vi "HTVacuumGUI.panel.vi"(0 "object ref":refnum<vi>, 5 "error in (no error)":errorcluster) -> (19 "error out":errorcluster)   [LabVIEW 2014, in "HTVacuumGUI.lvlib"]
doc: "This is just an example for a GUI thread.\n\nLicense Agreement for this software:\n\nCopyright (C)\nGesellschaft für Schwerionenforschung, GSI\nPlanckstr. 1\n64291 Darmstadt\nGermany\n\nContact: D.Beck@gsi.de \n\nThis program is free software; you can redistribute it and/or modify it under the terms of the GNU General Public License as published by the Free Software Foundation; either version 2 of the license, or (at your option) any later version.\n\nThis program is distributed in the hope that it will be useful, but WITHOUT ANYW ARRANTY; without even the implied warranty of MERCHANTABILITY or FITNESS FOR A PARTICULAR PURPOSE. See the GNU General License for more details (http://www.gnu.org).\n\nGesellschaft für Schwerionenforschung, GSI\nPlanckstr. 1, 64291 Darmstadt, Germany\nFor all questions and ideas contact: M.Richter@gsi.de, H.Brand@gsi.de or D.Beck@gsi.de.\nLast update: 18-DEC-2002"
uses:
  HTVacuumGUI.lvlib
  CS_Core/CSSystem/CoreLib/CoreLib.int 2 byte array.vi
  CS_Core/CSSystem/CoreLib/CoreLib.byte array 2 int.vi
  CS_Core/CSSystem/CoreLib/CoreLib.byte array 2 short.vi
  CS_Core/BaseProcess/BaseProcess.lvlib
  CS_Core/GUIs/GOGUserGUIs/DeviceBaseGUI/DeviceBaseGUI.lvlib
  CS_Core/CSSystem/CoreLib/CoreLib.lvlib
  CS_Core/CSSystem/CSSystemLib/CSSystemLib.lvlib
  CS_Core/CSObj/CSObj.lvlib
panel:
  in  "V62":bool
  out "V62":u32(colorbox)
  in  "V61":bool
  out "V61":u32(colorbox)
  in  "V52":bool
  out "V52":u32(colorbox)
  in  "V71":bool
  out "V71":u32(colorbox)
  in  "V1":bool
  out "V1":u32(colorbox)
  in  "VP3":bool
  out "VP3":u32(colorbox)
  in  "VP2":bool
  out "VP2":u32(colorbox)
  in  "VP1":bool
  out "VP1":u32(colorbox)
  in  "P3":bool
  out "P3":u32(colorbox)
  in  "P2":bool
  out "P2":u32(colorbox)
  in  "P1":bool
  out "P1":u32(colorbox)
  in  "SG 3VL":bool caption="Blank Button"
  in  "SG 2VL":bool caption="Blank Button"
  in  "SG 1VL":bool caption="Blank Button"
  in  "SG 3L":bool caption="Blank Button"
  in  "SG 2L":bool caption="Blank Button"
  in  "SG 1L":bool caption="Blank Button"
  in  "SP 3":bool caption="Blank Button"
  in  "SP 2":bool caption="Blank Button"
  out "G3":dbl(slide) scale=0.0..2.0
  out "G2":dbl(slide) scale=0.0..2.0
  out "G1":dbl(slide) scale=0.0..2.0
  in  "SP 1":bool caption="Blank Button"
  in  "stop":bool
  out "loop counter":i32
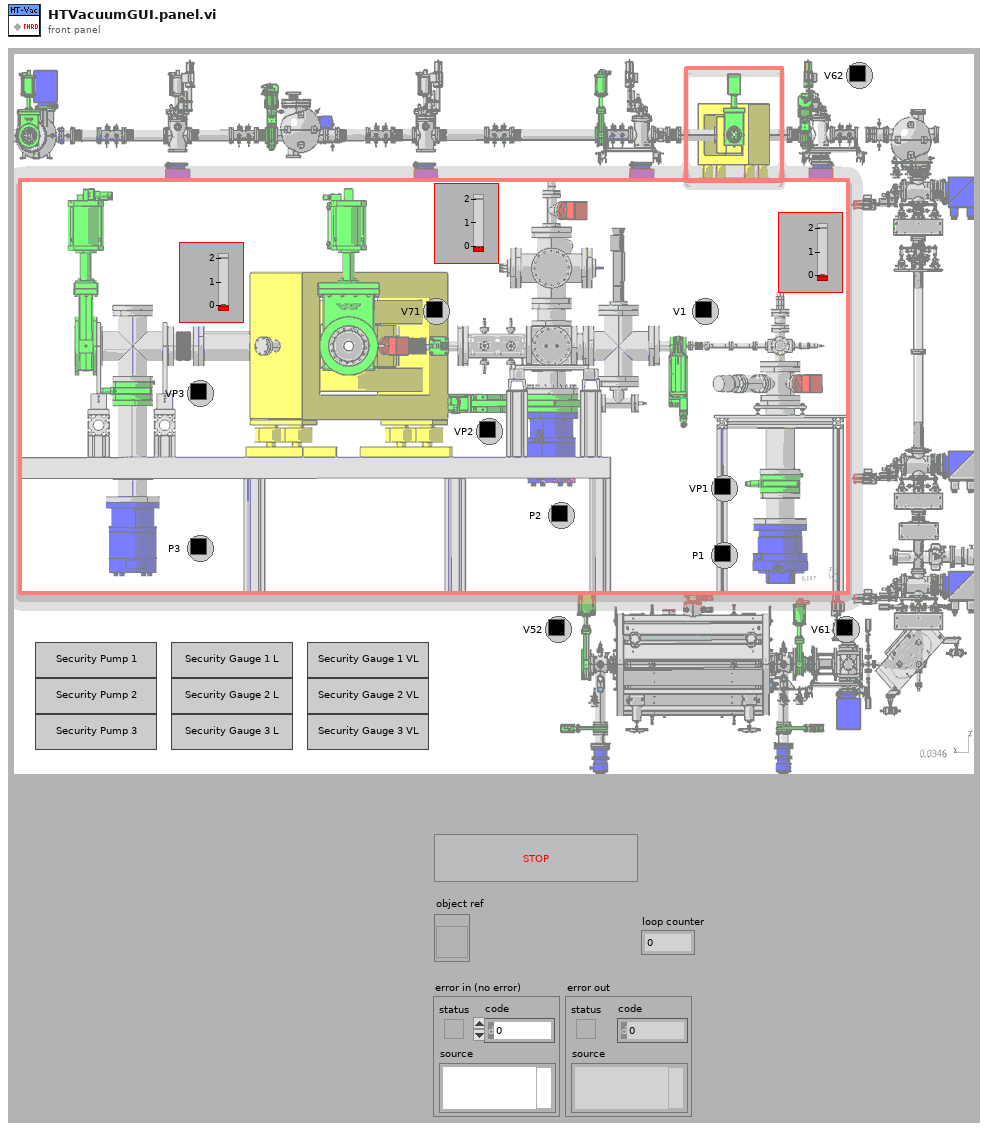
[diagram p1: front panel]
types:
  T1 = typedef "Semaphore RefNum" = refnum<k1>
  T2 = typedef "CoreDefs.rawDataType.ctl" = i8[]
  T3 = typedef "CoreDefs.call_type.ctl" = cluster{"Object":string, "Selector":string, "CallType":enum16{"simple", "synchronous", "asynchronous"}, "Async Object":string, "Async Selector":string, "Data Descriptor":T4, "Data":T2, "Error #":i32, "Expire":u32}
  T4 = typedef "BaseProcess.lvlib/BaseProcess.descriptor string definition.ctl" = string
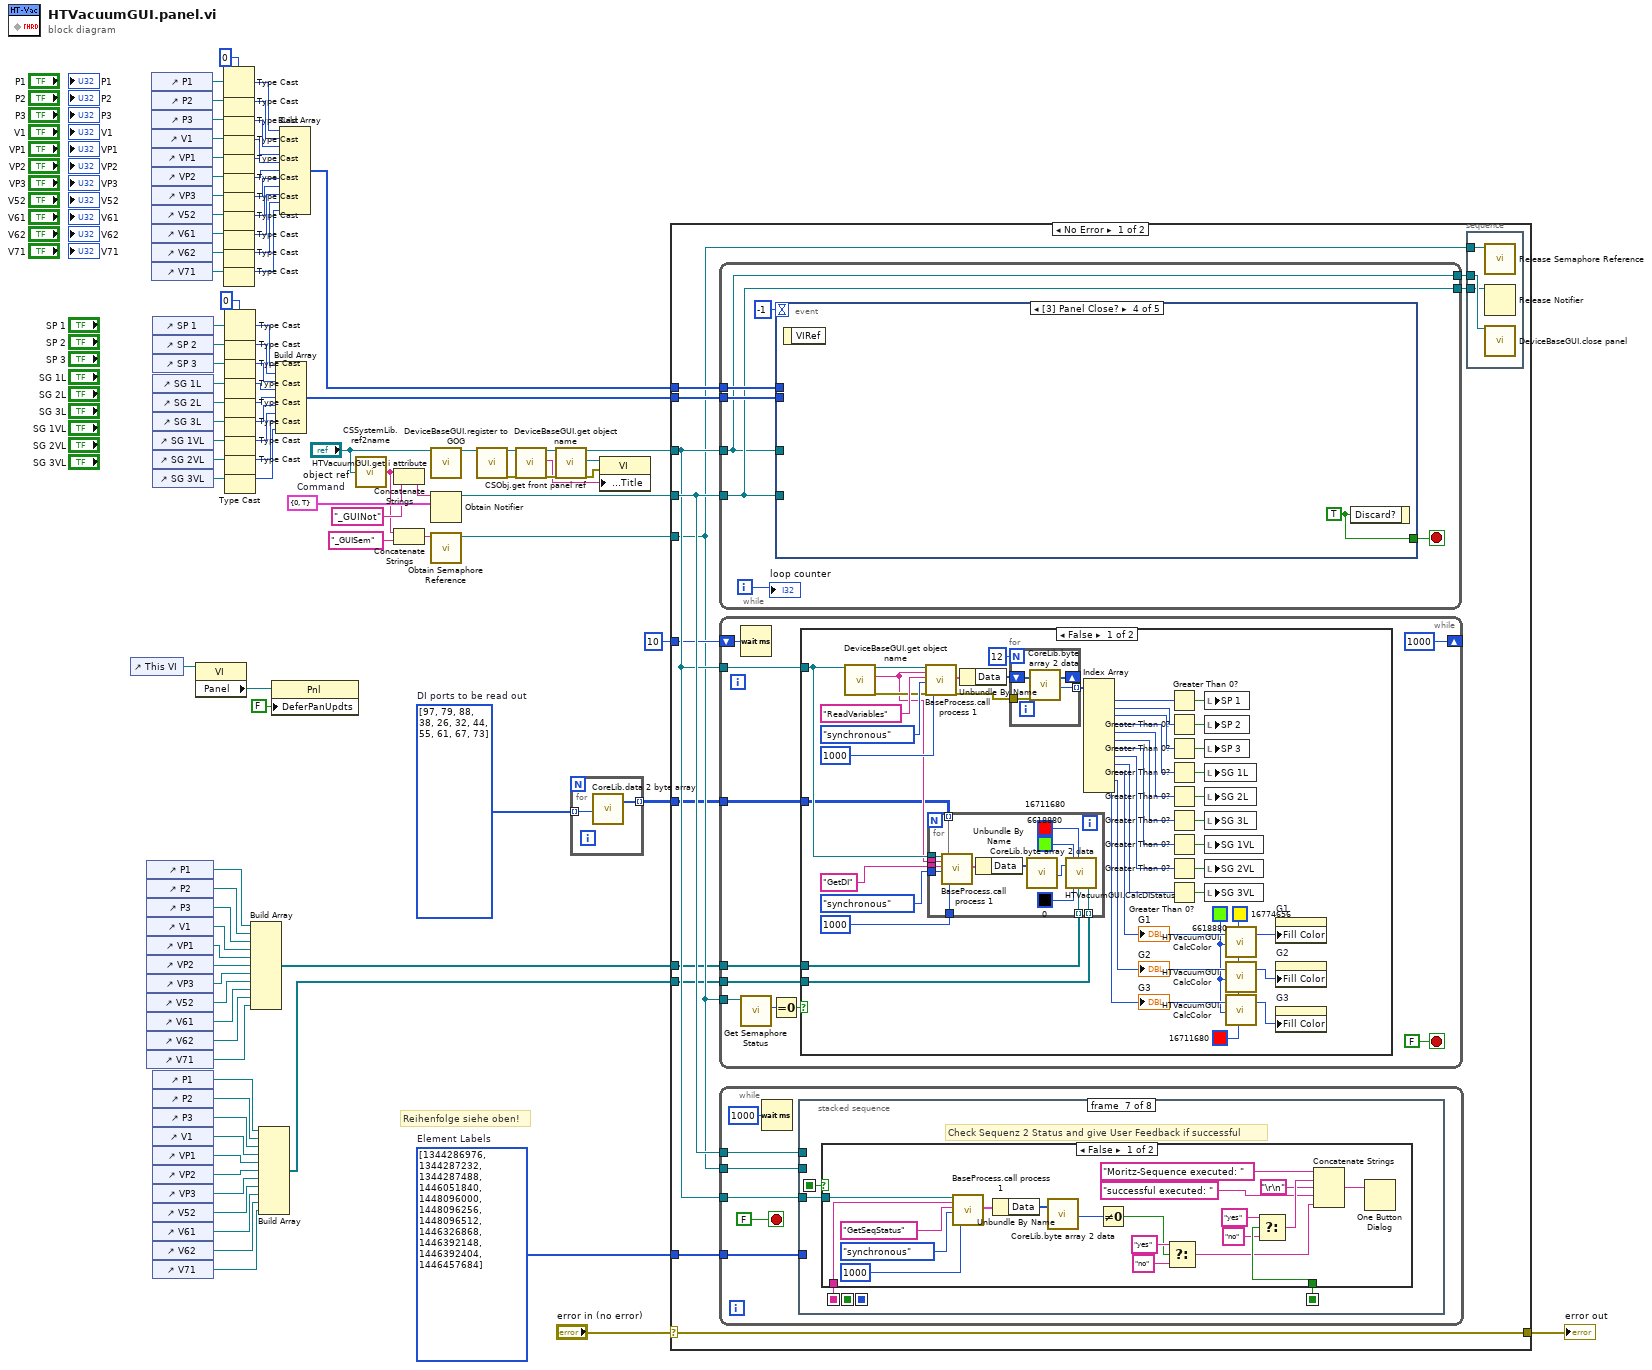
[diagram p0: block diagram]
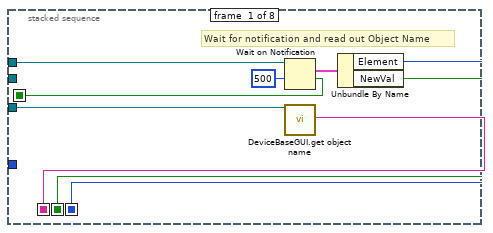
[diagram p2: hidden frame]
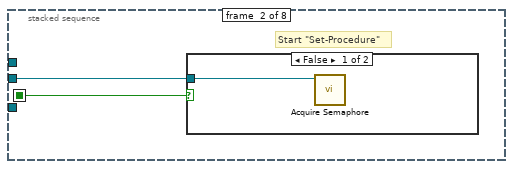
[diagram p3: hidden frame]
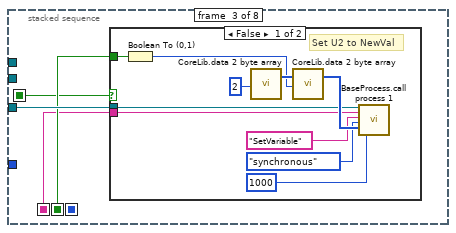
[diagram p5: hidden frame]
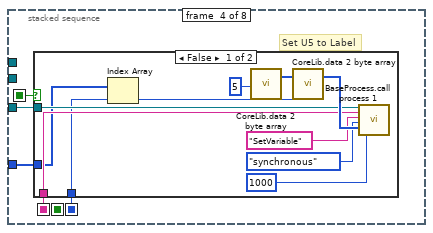
[diagram p7: hidden frame]
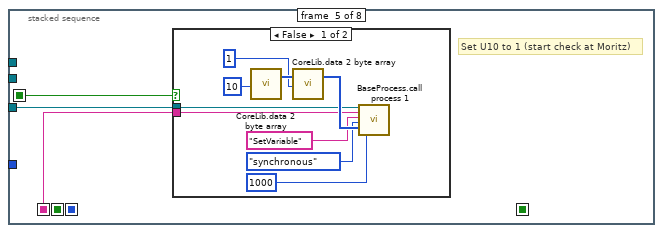
[diagram p9: hidden frame]
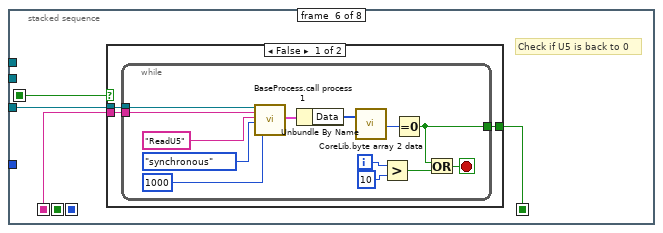
[diagram p11: hidden frame]
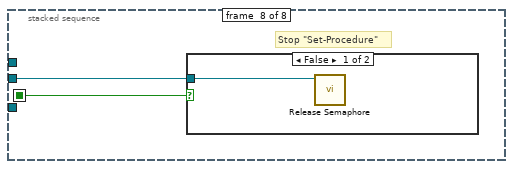
[diagram p14: hidden frame]
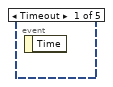
[diagram p17: hidden frame]
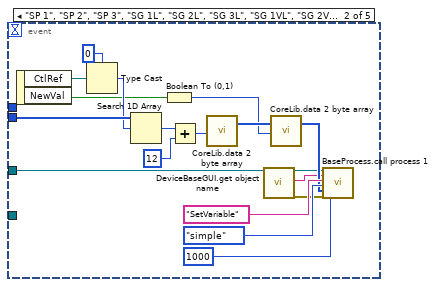
[diagram p18: hidden frame]
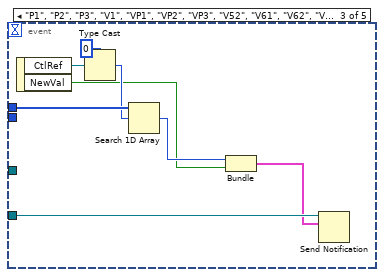
[diagram p19: hidden frame]
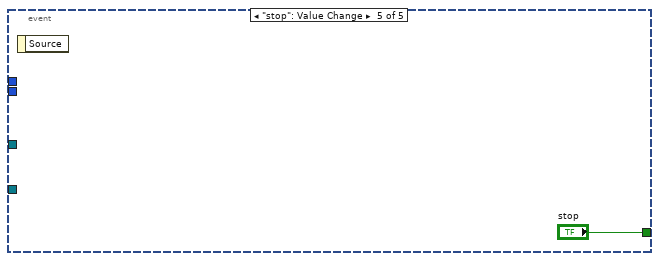
[diagram p20: hidden frame]
diagram:
  w29 = i32[] [97, 79, 88, 38, 26, 32, 44, 55, 61, 67, 73]  # DI ports to be read out
  w44 = i32[] [1344286976, 1344287232, 1344287488, 1446051840, 1448096000, 1448096256, 1448096512, 1446326868, 1446392148, 1446392404, 1446457684]  # Element Labels
  w49 = cluster{"Element":i32, "NewVal":bool} {"Element"=0, "NewVal"=TRUE}  # Command
  w51 = 0
  w84 = 0
  # "Reihenfolge siehe oben!"
  n1 = control-ref of="This VI"() -> (w3:refnum<vi>)
  n2 = control-ref of="P1"() -> (w27:refnum<vi>)
  n3 = control-ref of="P2"() -> (w26:refnum<vi>)
  n4 = control-ref of="P3"() -> (w25:refnum<vi>)
  n5 = control-ref of="V1"() -> (w24:refnum<vi>)
  n6 = control-ref of="VP1"() -> (w23:refnum<vi>)
  n7 = control-ref of="VP2"() -> (w22:refnum<vi>)
  n8 = control-ref of="VP3"() -> (w21:refnum<vi>)
  n9 = control-ref of="V52"() -> (w20:refnum<vi>)
  n10 = control-ref of="V61"() -> (w19:refnum<vi>)
  n11 = control-ref of="V62"() -> (w18:refnum<vi>)
  n12 = control-ref of="V71"() -> (w17:refnum<vi>)
  n13 = control-ref of="P1"() -> (w64:refnum<vi>)
  n14 = control-ref of="P2"() -> (w63:refnum<vi>)
  n15 = control-ref of="P3"() -> (w62:refnum<vi>)
  n16 = control-ref of="V1"() -> (w61:refnum<vi>)
  n17 = control-ref of="VP1"() -> (w60:refnum<vi>)
  n18 = control-ref of="VP2"() -> (w59:refnum<vi>)
  n19 = control-ref of="VP3"() -> (w58:refnum<vi>)
  n20 = control-ref of="V52"() -> (w57:refnum<vi>)
  n21 = control-ref of="V61"() -> (w56:refnum<vi>)
  n22 = control-ref of="V62"() -> (w55:refnum<vi>)
  n23 = control-ref of="V71"() -> (w54:refnum<vi>)
  n24 = control-ref of="SP 1"() -> (w93:refnum<vi>)
  n25 = control-ref of="SP 2"() -> (w92:refnum<vi>)
  n26 = control-ref of="SP 3"() -> (w91:refnum<vi>)
  n27 = control-ref of="SG 1L"() -> (w90:refnum<vi>)
  n28 = control-ref of="SG 2L"() -> (w89:refnum<vi>)
  n29 = control-ref of="SG 3L"() -> (w88:refnum<vi>)
  n30 = control-ref of="SG 1VL"() -> (w87:refnum<vi>)
  n31 = control-ref of="SG 2VL"() -> (w86:refnum<vi>)
  n32 = control-ref of="SG 3VL"() -> (w85:refnum<vi>)
  n33 = control-ref of="P1"() -> (w15:refnum<vi>)
  n34 = control-ref of="P2"() -> (w14:refnum<vi>)
  n35 = control-ref of="P3"() -> (w13:refnum<vi>)
  n36 = control-ref of="V1"() -> (w12:refnum<vi>)
  n37 = control-ref of="VP1"() -> (w11:refnum<vi>)
  n38 = control-ref of="VP2"() -> (w10:refnum<vi>)
  n39 = control-ref of="VP3"() -> (w9:refnum<vi>)
  n40 = control-ref of="V52"() -> (w8:refnum<vi>)
  n41 = control-ref of="V61"() -> (w7:refnum<vi>)
  n42 = control-ref of="V62"() -> (w6:refnum<vi>)
  n43 = control-ref of="V71"() -> (w5:refnum<vi>)
  n44 = property class="VI"(reference=w3) -> ("Panel"=w2:refnum<vi>)  [unwired: 1 in, 2 out]
  n45 = Type Cast(type=w51, x=w64) -> (*(type *) &x=w73:i32)
  n46 = Type Cast(type=w51, x=w63) -> (*(type *) &x=w72:i32)
  n47 = Type Cast(type=w51, x=w62) -> (*(type *) &x=w71:i32)
  n48 = Type Cast(type=w51, x=w61) -> (*(type *) &x=w70:i32)
  n49 = Type Cast(type=w51, x=w60) -> (*(type *) &x=w69:i32)
  n50 = Type Cast(type=w51, x=w59) -> (*(type *) &x=w68:i32)
  n51 = Type Cast(type=w51, x=w58) -> (*(type *) &x=w67:i32)
  n52 = Type Cast(type=w51, x=w57) -> (*(type *) &x=w66:i32)
  n53 = Type Cast(type=w51, x=w56) -> (*(type *) &x=w65:i32)
  n54 = Type Cast(type=w51, x=w55) -> (*(type *) &x=w53:i32)
  n55 = Type Cast(type=w51, x=w54) -> (*(type *) &x=w52:i32)
  n56 = Type Cast(type=w84, x=w93) -> (*(type *) &x=w83:i32)
  n57 = Type Cast(type=w84, x=w92) -> (*(type *) &x=w82:i32)
  n58 = Type Cast(type=w84, x=w91) -> (*(type *) &x=w81:i32)
  n59 = Type Cast(type=w84, x=w90) -> (*(type *) &x=w80:i32)
  n60 = Type Cast(type=w84, x=w89) -> (*(type *) &x=w79:i32)
  n61 = Type Cast(type=w84, x=w88) -> (*(type *) &x=w78:i32)
  n62 = Type Cast(type=w84, x=w87) -> (*(type *) &x=w77:i32)
  n63 = Type Cast(type=w84, x=w86) -> (*(type *) &x=w76:i32)
  n64 = Type Cast(type=w84, x=w85) -> (*(type *) &x=w75:i32)
  n65 = Build Array(w27, w26, w25, w24, w23, w22, w21, w20, w19, w18, w17) -> (w16:refnum<vi>[])
  n66 = Build Array(w15, w14, w13, w12, w11, w10, w9, w8, w7, w6, w5) -> (w4:refnum<vi>[])
  n67 = property class="Pnl"(reference=w2, "DeferPanUpdts"=FALSE ("Defer Panel Updates")) -> ()  [unwired: 1 in, 2 out]
  n68 = Build Array(w83, w82, w81, w80, w79, w78, w77, w76, w75) -> (w74:i32[])
  n69 = Build Array(w73, w72, w71, w70, w69, w68, w67, w66, w65, w53, w52) -> (w50:i32[])
  n70 = call "CSSystemLib.ref2name.vi"("obj refnum"="object ref") -> ("name"=w42:string)
  n71 = Concatenate Strings(w42, "_GUINot" ("string")) -> (w47:string)
  n72 = Concatenate Strings(w42, "_GUISem" ("string")) -> (w43:string)
  n73 = call "HTVacuumGUI.get i attribute.vi"("i ref in"="object ref") -> ("i ref out"=w32:refnum<vi>)  [unwired: 16 in, 2 out]
  n74 = Obtain Notifier(name (unnamed)=w47, notification data type=w49) -> (notifier out=w45:refnum<notifier>)  [unwired: 2 in, 2 out]
  n75 = call <vilib>:"Obtain Semaphore Reference.vi"("name (unnamed)"=w43) -> ("semaphore"=w40:T1)  [unwired: 4 in, 2 out]
  n76 = call "DeviceBaseGUI.register to GOG.vi"("i ref in"=w32) -> ("i ref out"=w37:refnum<vi>, "error out"=w38:errorcluster)  [unwired: 16 in, 1 out]
  n77 = call "DeviceBaseGUI.get object name.vi"("i ref in"=w37, "error in (no error)"=w38) -> ("i ref out"=w36:refnum<vi>, "objectName"=w33:string, "error out"=w35:errorcluster)  [unwired: 15 in]
  n78 = call "CSObj.get front panel ref.vi"("i ref in"=w36, "error in (no error)"=w35) -> ("i ref out"=w31:refnum<vi>, "frontPanelRef"=w39:refnum<vi>, "error out"=w34:errorcluster)  [unwired: 15 in]
  n79 = for {
    tunnel: w29 -> [w97] mode=indexing
    tunnel: [w96] -> w28 mode=indexing
    n80 = call-poly "CoreLib.data 2 byte array.vi"("i32"=w97) -> ("byteArray out"=w96:T2)  [unwired: 18 in]
  }
  n81 = property class="VI"(reference=w39, error in=w34, "Front Panel Window:Title"=w33) -> ()  [unwired: 2 out]
  n82 = case shown="No Error" "error in (no error)" {
    selector: "error in (no error)" -> [w110 w331]
    tunnel: [w110 w331] -> w94
    tunnel: w31 -> [w106 w330]
    tunnel: w74 -> [w109 _]
    tunnel: w50 -> [w108 _]
    tunnel: w45 -> [w107 w328]
    tunnel: w44 -> [w105 _]
    tunnel: w40 -> [w101 w329]
    tunnel: 10 -> [w104 _]
    tunnel: w28 -> [w100 _]
    tunnel: w16 -> [w99 _]
    tunnel: w4 -> [w98 _]
    frame No Error {
      n83 = while {
        tunnel: w106 -> [w293]
        tunnel: w109 -> [w296]
        tunnel: w108 -> [w295]
        tunnel: w107 -> [w294]
        tunnel: [w294] -> w102
        tunnel: [w293] -> w103
        i -> [w298]
        stop <- w299 stop-if-true
        n84 = event shown="[3] Panel Close?" {
          selector: _ -> [_ _ _ _ _]
          dyn-events: _ -> [_ _ _ _ _]
          timeout: -1 -> [_ _ _ _ _]
          tunnel: [_ _ _ w326 "stop"] -> w299
          tunnel: w293 -> [_ w301 _ _ _]
          tunnel: w296 -> [_ w315 _ _ _]
          tunnel: w295 -> [_ _ w323 _ _]
          tunnel: w294 -> [_ _ w321 _ _]
          event Timeout {
            n85 = event-data() -> ()  [unwired: 1 in, 1 out]
          }
          event "SP 1", "SP 2", "SP 3", "SG 1L", "SG 2L", "SG 3L", "SG 1VL", "SG 2VL", "SG 3VL": Value Change {
            n86 = event-data() -> ("CtlRef"=w316:refnum<vi>, "NewVal"=w308:bool)  [unwired: 1 in]
            n87 = Type Cast(type=0, x=w316) -> (*(type *) &x=w314:i32)
            n88 = Search 1D Array(1D array=w315, element=w314) -> (index of element=w305:i32)  [unwired: 1 in]
            n89 = Boolean To (0,1)(Boolean=w308) -> (0, 1=w307:i16)
            n90 = Add(x=w305, y=12) -> (x+y=w306:i32)
            n91 = call-poly "CoreLib.data 2 byte array.vi"("i32"=w306) -> ("byteArray out"=w309:T2)  [unwired: 18 in]
            n92 = call "DeviceBaseGUI.get object name.vi"("i ref in"=w301) -> ("i ref out"=w302:refnum<vi>, "objectName"=w300:string, "error out"=w303:errorcluster)  [unwired: 16 in]
            n93 = call-poly "CoreLib.data 2 byte array.vi"("byteArray"=w309, "i32"=w307) -> ("byteArray out"=w310:T2)  [unwired: 17 in]
            n94 = call "BaseProcess.call process 1.vi"("i ref in"=w302, "Object"=w300, "Selector"="SetVariable", "CallType"=enum16{"simple", "synchronous", "asynchronous"}."simple", "Data"=w310, "error in (no error)"=w303, "timeout (ms)"=1000) -> ()  [unwired: 10 in, 3 out]
          }
          event "P1", "P2", "P3", "V1", "VP1", "VP2", "VP3", "V52", "V61", "V62", "V71": Value Change {
            n95 = event-data() -> ("CtlRef"=w324:refnum<vi>, "NewVal"=w319:bool)  [unwired: 1 in]
            n96 = Type Cast(type=0, x=w324) -> (*(type *) &x=w322:i32)
            n97 = Search 1D Array(1D array=w323, element=w322) -> (index of element=w320:i32)  [unwired: 1 in]
            n98 = Bundle("index of element"=w320, "NewVal"=w319) -> (w318:cluster{"index of element":i32, "NewVal":bool})  [unwired: 1 in]
            n99 = Send Notification(notification=w318, notifier=w321) -> ()  [unwired: 1 in, 2 out]
          }
          event Panel Close? {
            w326 = TRUE ("Discard?")
            n100 = event-data() -> ()  [unwired: 1 in, 1 out]
            n101 = event-data("Discard?"=w326) -> ()  [unwired: 1 in, 1 out]
          }
          event "stop": Value Change {
            n102 = event-data() -> ()  [unwired: 1 in, 1 out]
          }
        }
        "loop counter" <- w298
      }
      n103 = while {
        tunnel: w106 -> [w229]
        tunnel: w101 -> [w226]
        shift-right: [1000 ("ms timeout (-1)")] -> _
        shift-left: w104 -> [w223]
        tunnel: w100 -> [w222]
        tunnel: w99 -> [w221]
        tunnel: w98 -> [w220]
        stop <- FALSE stop-if-true
        n104 = Wait (ms)(milliseconds to wait=w223) -> ()  [unwired: 1 out]
        n105 = call <vilib>:"Get Semaphore Status.vi"("semaphore"=w226) -> ("# available"=w228:i32)  [unwired: 5 in, 5 out]
        n106 = Equal To 0?(x=w228) -> (x = 0?=w227:bool)
        n107 = case shown="False" w227 {
          tunnel: w229 -> [w237 _]
          tunnel: w222 -> [w232 _]
          tunnel: w221 -> [w231 _]
          tunnel: w220 -> [w230 _]
          frame False {
            w241 = u32 16711680
            w242 = u32 16774656
            w240 = u32 6618880
            n108 = call "DeviceBaseGUI.get object name.vi"("i ref in"=w237) -> ("i ref out"=w248:refnum<vi>, "objectName"=w236:string, "error out"=w247:errorcluster)  [unwired: 16 in]
            n109 = call "BaseProcess.call process 1.vi"("i ref in"=w248, "Object"=w236, "Selector"="ReadVariables", "CallType"=enum16{"simple", "synchronous", "asynchronous"}."synchronous", "error in (no error)"=w247, "timeout (ms)"=1000) -> ("call cluster out"=w271:T3, "error out"=w268:errorcluster)  [unwired: 11 in, 1 out]
            n110 = for {
              tunnel: w237 -> [w288]
              tunnel: w236 -> [w287]
              tunnel: "GetDI" ("Selector") -> [w286]
              tunnel: enum16{"simple", "synchronous", "asynchronous"}."synchronous" ("CallType") -> [w285]
              tunnel: 1000 ("timeout (ms)") -> [w284]
              tunnel: w232 -> [w283] mode=indexing
              tunnel: w231 -> [w279] mode=indexing
              tunnel: w230 -> [w275] mode=indexing
              n111 = call "BaseProcess.call process 1.vi"("i ref in"=w288, "Object"=w287, "Selector"=w286, "CallType"=w285, "Data"=w283, "timeout (ms)"=w284) -> ("call cluster out"=w282:T3)  [unwired: 11 in, 2 out]
              n112 = Unbundle By Name(w282) -> ("Data"=w281:T2)
              n113 = call-poly "CoreLib.byte array 2 data.vi"("byteArray"=w281) -> ("i16"=w280:i16)  [unwired: 16 in, 2 out]
              n114 = call "HTVacuumGUI.CalcDIStatus.vi"("DIStatus"=w280, "Color2"=u32 6618880, "Color3"=u32 0, "Color1"=u32 16711680, "Color Control Ref"=w279, "Boolen Ref"=w275) -> ()  [unwired: 14 in]
            }
            n115 = Unbundle By Name(w271) -> ("Data"=w270:T2)
            n116 = for {
              N: 12 -> [_]
              shift-right: [w291] -> _
              shift-left: w270 -> [w292]
              tunnel: w268 -> [w290]
              tunnel: [w289] -> w258 mode=indexing
              n117 = call-poly "CoreLib.byte array 2 data.vi"("byteArray"=w292, "error in (no error)"=w290) -> ("byteArray out"=w291:T2, "i32"=w289:i32)  [unwired: 15 in, 1 out]
            }
            n118 = Index Array(array=w258) -> (element #1=w267:i32, element #2=w266:i32, element #3=w265:i32, element #4=w264:i32, element #5=w263:i32, element #6=w262:i32, element #7=w261:i32, element #8=w260:i32, element #9=w259:i32, element #10=w246:i32, element #11=w244:i32, element #12=w243:i32)  [unwired: 12 in]
            "G1" <- w246
            "G2" <- w244
            "G3" <- w243
            n119 = Greater Than 0?(x=w267) -> (x > 0?=w257:bool)
            n120 = Greater Than 0?(x=w266) -> (x > 0?=w256:bool)
            n121 = Greater Than 0?(x=w265) -> (x > 0?=w255:bool)
            n122 = Greater Than 0?(x=w264) -> (x > 0?=w254:bool)
            n123 = Greater Than 0?(x=w263) -> (x > 0?=w253:bool)
            n124 = Greater Than 0?(x=w262) -> (x > 0?=w252:bool)
            n125 = Greater Than 0?(x=w261) -> (x > 0?=w251:bool)
            n126 = Greater Than 0?(x=w260) -> (x > 0?=w250:bool)
            n127 = Greater Than 0?(x=w259) -> (x > 0?=w249:bool)
            n128 = local write "SP 1"(w257) -> ()
            n129 = local write "SP 2"(w256) -> ()
            n130 = local write "SP 3"(w255) -> ()
            n131 = local write "SG 1L"(w254) -> ()
            n132 = local write "SG 2L"(w253) -> ()
            n133 = local write "SG 3L"(w252) -> ()
            n134 = local write "SG 1VL"(w251) -> ()
            n135 = local write "SG 2VL"(w250) -> ()
            n136 = local write "SG 3VL"(w249) -> ()
            n137 = call "HTVacuumGUI.CalcColor.vi"("Input-Value"=w246, "Color1"=w240, "Color2"=w242, "Color3"=w241) -> ("Output-Value"=w245:u32)  [unwired: 15 in]
            n138 = call "HTVacuumGUI.CalcColor.vi"("Input-Value"=w244, "Color1"=w240, "Color2"=w242, "Color3"=w241) -> ("Output-Value"=w239:u32)  [unwired: 15 in]
            n139 = call "HTVacuumGUI.CalcColor.vi"("Input-Value"=w243, "Color1"=w240, "Color2"=w242, "Color3"=w241) -> ("Output-Value"=w238:u32)  [unwired: 15 in]
            n140 = property on="G1" class="Slide (strict)"("Fill Color"=w245) -> ()  [unwired: 2 in, 2 out]
            n141 = property on="G2" class="Slide (strict)"("Fill Color"=w239) -> ()  [unwired: 2 in, 2 out]
            n142 = property on="G3" class="Slide (strict)"("Fill Color"=w238) -> ()  [unwired: 2 in, 2 out]
          }
          frame True {
          }
        }
      }
      n143 = while {
        tunnel: w107 -> [w119]
        tunnel: w106 -> [w118]
        tunnel: w105 -> [w117]
        tunnel: w101 -> [w116]
        stop <- FALSE stop-if-true
        n144 = Wait (ms)(milliseconds to wait=u32 1000) -> ()  [unwired: 1 out]
        n145 = stacked-sequence {
          seq-local: [w120 _ _ _ _ _ _ _] -> [_ _ w132 w148 w162 w175 w195 _]
          seq-local: [w124 _ _ _ _ _ _ _] -> [_ _ w133 _ _ _ _ _]
          seq-local: [w125 _ _ _ _ _ _ _] -> [_ _ _ w147 _ _ _ _]
          seq-local: [_ _ _ _ _ w174 _ _] -> [_ _ _ _ _ _ w194 _]
          seq-local: [w122 _ _ _ _ _ _ _] -> [_ w129 w131 w146 w161 w173 w193 w218]
          tunnel: w119 -> [w127 _ _ _ _ _ _ _]
          tunnel: w118 -> [w121 _ w134 w149 w163 w176 w196 _]
          tunnel: w117 -> [_ _ _ w145 _ _ _ _]
          tunnel: w116 -> [_ w128 _ _ _ _ _ w217]
          frame #0 {
            # "Wait for notification and read out Object Name"
            n146 = Wait on Notification(notifier=w127, timeout in ms (-1)=500) -> (notification=w126:cluster{"Element":i32, "NewVal":bool}, timed out?=w122:bool)  [unwired: 2 in, 2 out]
            n147 = call "DeviceBaseGUI.get object name.vi"("i ref in"=w121) -> ("objectName"=w120:string)  [unwired: 16 in, 2 out]
            n148 = Unbundle By Name(w126) -> ("Element"=w125:i32, "NewVal"=w124:bool)
          }
          frame #1 {
            # "Start \"Set-Procedure\""
            n149 = case shown="False" w129 {
              tunnel: w128 -> [w130 _]
              frame False {
                n150 = call <vilib>:"Acquire Semaphore.vi"("semaphore"=w130) -> ()  [unwired: 4 in, 3 out]
              }
              frame True {
              }
            }
          }
          frame #2 {
            n151 = case shown="False" w131 {
              tunnel: w134 -> [w138 _]
              tunnel: w133 -> [w137 _]
              tunnel: w132 -> [w135 _]
              frame False {
                # "Set U2 to NewVal"
                n152 = Boolean To (0,1)(Boolean=w137) -> (0, 1=w136:i16)
                n153 = call-poly "CoreLib.data 2 byte array.vi"("i32"=2) -> ("byteArray out"=w143:T2)  [unwired: 18 in]
                n154 = call-poly "CoreLib.data 2 byte array.vi"("byteArray"=w143, "i32"=w136) -> ("byteArray out"=w144:T2)  [unwired: 17 in]
                n155 = call "BaseProcess.call process 1.vi"("i ref in"=w138, "Object"=w135, "Selector"="SetVariable", "CallType"=enum16{"simple", "synchronous", "asynchronous"}."synchronous", "Data"=w144, "timeout (ms)"=1000) -> ()  [unwired: 11 in, 3 out]
              }
              frame True {
              }
            }
          }
          frame #3 {
            # "Set U5 to Label"
            n156 = case shown="False" w146 {
              tunnel: w149 -> [w154 _]
              tunnel: w148 -> [w153 _]
              tunnel: w147 -> [w152 _]
              tunnel: w145 -> [w150 _]
              frame False {
                n157 = Index Array(array=w150, index=w152) -> (element=w151:i32)
                n158 = call-poly "CoreLib.data 2 byte array.vi"("i32"=5) -> ("byteArray out"=w159:T2)  [unwired: 18 in]
                n159 = call-poly "CoreLib.data 2 byte array.vi"("byteArray"=w159, "i32"=w151) -> ("byteArray out"=w160:T2)  [unwired: 17 in]
                n160 = call "BaseProcess.call process 1.vi"("i ref in"=w154, "Object"=w153, "Selector"="SetVariable", "CallType"=enum16{"simple", "synchronous", "asynchronous"}."synchronous", "Data"=w160, "timeout (ms)"=1000) -> ()  [unwired: 11 in, 3 out]
              }
              frame True {
              }
            }
          }
          frame #4 {
            # "Set U10 to 1 (start check at Moritz)"
            n161 = case shown="False" w161 {
              tunnel: w163 -> [w166 _]
              tunnel: w162 -> [w165 _]
              frame False {
                n162 = call-poly "CoreLib.data 2 byte array.vi"("i32"=10) -> ("byteArray out"=w171:T2)  [unwired: 18 in]
                n163 = call-poly "CoreLib.data 2 byte array.vi"("byteArray"=w171, "i32"=1) -> ("byteArray out"=w172:T2)  [unwired: 17 in]
                n164 = call "BaseProcess.call process 1.vi"("i ref in"=w166, "Object"=w165, "Selector"="SetVariable", "CallType"=enum16{"simple", "synchronous", "asynchronous"}."synchronous", "Data"=w172, "timeout (ms)"=1000) -> ()  [unwired: 11 in, 3 out]
              }
              frame True {
              }
            }
          }
          frame #5 {
            # "Check if U5 is back to 0"
            n165 = case shown="False" w173 {
              tunnel: w176 -> [w179 _]
              tunnel: w175 -> [w178 _]
              tunnel: [w177 _] -> w174
              frame False {
                n166 = while {
                  tunnel: w179 -> [w189]
                  tunnel: w178 -> [w188]
                  tunnel: [w182] -> w177
                  i -> [w184]
                  stop <- w181 stop-if-true
                  n167 = call "BaseProcess.call process 1.vi"("i ref in"=w189, "Object"=w188, "Selector"="ReadU5", "CallType"=enum16{"simple", "synchronous", "asynchronous"}."synchronous", "timeout (ms)"=1000) -> ("call cluster out"=w187:T3)  [unwired: 12 in, 2 out]
                  n168 = Unbundle By Name(w187) -> ("Data"=w186:T2)
                  n169 = call-poly "CoreLib.byte array 2 data.vi"("byteArray"=w186) -> ("i32"=w185:i32)  [unwired: 16 in, 2 out]
                  n170 = Greater?(x=w184, y=10) -> (0:w180:bool)
                  n171 = Equal To 0?(x=w185) -> (x = 0?=w182:bool)
                  n172 = Or(x=w182, y=w180) -> (x .or. y?=w181:bool)
                }
              }
              frame True {
              }
            }
          }
          frame #6 {
            # "Check Sequenz 2 Status and give User Feedback if successful"
            n173 = case shown="False" w193 {
              tunnel: w196 -> [w213 _]
              tunnel: w195 -> [w212 _]
              tunnel: w194 -> [w208 _]
              frame False {
                n174 = call "BaseProcess.call process 1.vi"("i ref in"=w213, "Object"=w212, "Selector"="GetSeqStatus", "CallType"=enum16{"simple", "synchronous", "asynchronous"}."synchronous", "timeout (ms)"=1000) -> ("call cluster out"=w211:T3)  [unwired: 12 in, 2 out]
                n175 = Unbundle By Name(w211) -> ("Data"=w210:T2)
                n176 = call-poly "CoreLib.byte array 2 data.vi"("byteArray"=w210) -> ("i16"=w199:i16)  [unwired: 16 in, 2 out]
                n177 = Not Equal To 0?(x=w199) -> (x != 0?=w198:bool)
                n178 = Select(t="yes", s=w198, f="no") -> (s? t:f=w200:string)
                n179 = Select(t="yes", s=w208, f="no") -> (s? t:f=w207:string)
                n180 = Concatenate Strings("Moritz-Sequence executed: ", w207, "\r\n", "successful executed: ", w200) -> (w197:string)
                n181 = One Button Dialog(message=w197) -> ()  [unwired: 1 in, 1 out]
              }
              frame True {
              }
            }
          }
          frame #7 {
            # "Stop \"Set-Procedure\""
            n182 = case shown="False" w218 {
              tunnel: w217 -> [w219 _]
              frame False {
                n183 = call <vilib>:"Release Semaphore.vi"("semaphore"=w219) -> ()  [unwired: 5 in, 2 out]
              }
              frame True {
              }
            }
          }
        }
      }
      n184 = stacked-sequence {
        tunnel: w103 -> [w113]
        tunnel: w102 -> [w112]
        tunnel: w101 -> [w111]
        frame #0 {
          n185 = call <vilib>:"Release Semaphore Reference.vi"("semaphore"=w111) -> ()  [unwired: 9 in, 2 out]
          n186 = Release Notifier(notifier=w112) -> ()  [unwired: 2 in, 3 out]
          n187 = call "DeviceBaseGUI.close panel.vi"("i ref in"=w113) -> ()  [unwired: 17 in, 2 out]
        }
      }
    }
    frame Error {
      n188 = call "DeviceBaseGUI.close panel.vi"("i ref in"=w330) -> ()  [unwired: 17 in, 2 out]
      n189 = Release Notifier(notifier=w328) -> ()  [unwired: 2 in, 3 out]
      n190 = call <vilib>:"Release Semaphore Reference.vi"("semaphore"=w329) -> ()  [unwired: 9 in, 2 out]
    }
  }
  "error out" <- w94
